vi "CVT2BasicInit.vi"() -> (0 "error out":errorcluster, 2 "Tags per type out":i32, 3 "names":string[](array[string]))   [LabVIEW 2014, in "UnitTests.lvlib"]
uses:
  UnitTests.lvlib
  dev/source/vi.lib/NI/Current Value Table/Current Value Table.lvlib
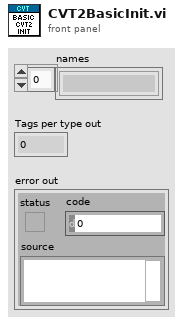
[diagram p1: front panel]
types:
  T1 = typedef "Current Value Table.lvlib/File Format.ctl" = cluster{"Tags":T2[], "Group Listings":T4[]}
  T2 = typedef "Current Value Table.lvlib/Single Tag.ctl" = cluster{"Data Type":T3, "Name":string, "Value":string, "Description":string}
  T3 = typedef "Current Value Table.lvlib/Data Types.ctl" = enum16{"Double", "Single", "I64", "I32", "I16", "I8", "U64", "U32", "U16", "U8", "String", "Boolean", "Array of U8", "Array of U16", "Array of U32", "Array of U64", "Array of I64", "Array of I32", "Array of I16", "Array of I8", "Array of Double", "Array of Single", "Array of Boolean", "Array of String"}
  T4 = typedef "Current Value Table.lvlib/Tag Grouping set.ctl" = cluster{"Group":string, "Tag Names":string[]}
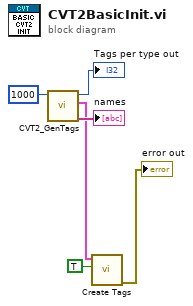
[diagram p0: block diagram]
diagram:
  n1 = call "CVT2_GenTags.vi"("Tags per type"=1000 ("Number of Tags in")) -> ("names"=→"names":string[], "Init data"=w1:T1, "Tags per type out"=→"Tags per type out":i32)  [unwired: 7 in, 1 out]
  n2 = call "Create Tags.vi"("Clear Table? (F)"=TRUE, "CVT Tags to Create"=w1) -> ("error out"=→"error out":errorcluster)  [unwired: 9 in]
